vi "create key.vi"(11 "data dictionary in":refnum<class "data dictionary.lvclass">) -> (3 "key":string)   [LabVIEW 2013, in "TEC runtime.lvclass"]
uses:
  TEC runtime.lvclass
  <vilib>/NI/Tag Bus/dictionary/data dictionary.lvclass
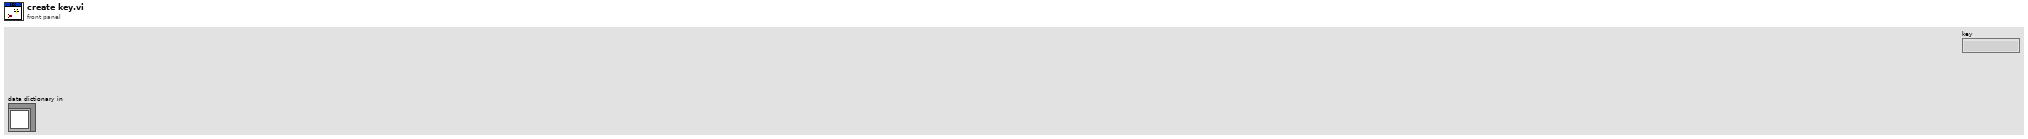
[diagram p1: front panel]
types:
  T1 = typedef "tag bus.lvlib/data table.lvlib/allocation specification.ctl" = cluster{"data type":T2, "size":i32}
  T2 = typedef "tag bus.lvlib/tag descriptor.lvclass/Data Type.ctl" = enum16{"Double", "Single", "I64", "I32", "I16", "I8", "U64", "U32", "U16", "U8", "Boolean", "String", "Array of Double", "Array of Single", "Array of I64", "Array of I32", "Array of I16", "Array of I8", "Array of U64", "Array of U32", "Array of U16", "Array of U8", "Array of Boolean", "Array of String"}
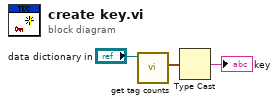
[diagram p0: block diagram]
diagram:
  n1 = call <vilib>:"get tag counts.vi"("data dictionary in"="data dictionary in") -> ("counts"=w2:T1[])  [unwired: 9 in, 1 out]
  n2 = Type Cast(x=w2) -> (*(type *) &x=→"key":string)  [unwired: 1 in]
